vi "Start Receiving.vi"(8 "error in (no error)":errorcluster, 10 "Input":T1, 11 "Vision in":refnum<class "Vision.lvclass">) -> (0 "error out":errorcluster, 3 "Vision out":refnum<class "Vision.lvclass">)   [LabVIEW 2022 SP3, in "Vision.lvlib" / "Vision.lvclass"]
uses:
  UDP Input.ctl
  Vision.lvclass
  Vision.lvclass/Vision.ctl
  UDP Data Receiver/UDP Data Receiver Messages/Start Receiving Msg/Start Receiving Msg.lvclass
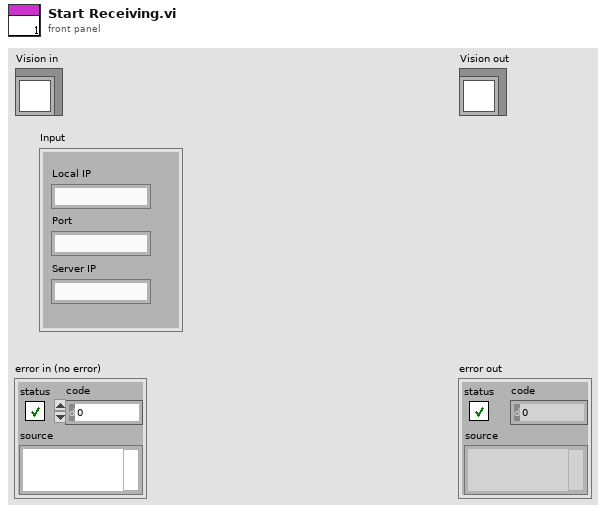
[diagram p1: front panel]
types:
  T1 = typedef "UDP Input.ctl" = cluster{"Local IP":string, "Port":string, "Server IP":string}
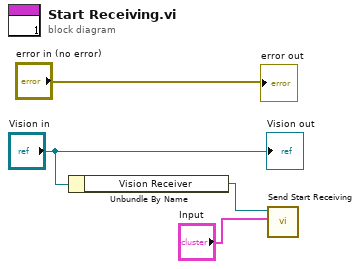
[diagram p0: block diagram]
diagram:
  n1 = Unbundle By Name("Vision in") -> ("Vision Receiver"=w1:refnum<class "Message Enqueuer.lvclass">)
  n2 = call "Send Start Receiving.vi"("Input"="Input", "Message Enqueuer"=w1) -> ()  [unwired: 8 in, 2 out]
  "error out" <- "error in (no error)"
  "Vision out" <- "Vision in"
